vi "DataLib.pack data.vi"(1 "dataIn":T1, 2 "DAQDevice":string, 3 "Data Descriptor":T2, 4 "DAQDeviceData":T1) -> (15 "dataOut":T1)   [LabVIEW 2014, in "DataLib.lvlib"]
doc: "Packs the data of each DAQ device by the EventBuilder class."
uses:
  DataLib.lvlib
  CSCore/CSSystem/CoreDefs/CoreDefs.rawDataType.ctl
  CSCore/BaseProcess/BaseProcess.descriptor string definition.ctl
  CSCore/CSSystem/CoreLib/CoreLib.string 2 byte array.vi
  CSCore/CSSystem/CoreLib/CoreLib.lvlib
  CSCore/BaseProcess/BaseProcess.lvlib
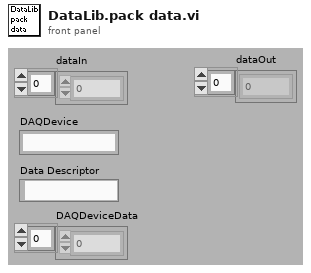
[diagram p1: front panel]
types:
  T1 = typedef "CoreDefs.rawDataType.ctl" = i8[]
  T2 = typedef "BaseProcess.lvlib/BaseProcess.descriptor string definition.ctl" = string
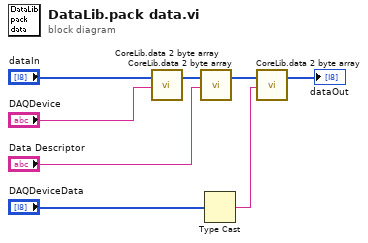
[diagram p0: block diagram]
diagram:
  n1 = call-poly "CoreLib.data 2 byte array.vi"("byteArray"="dataIn", "string"="DAQDevice") -> ("byteArray out"=w7:T1)  [unwired: 17 in]
  n2 = call-poly "CoreLib.data 2 byte array.vi"("byteArray"=w7, "string"="Data Descriptor") -> ("byteArray out"=w4:T1)  [unwired: 17 in]
  n3 = Type Cast(x="DAQDeviceData") -> (*(type *) &x=w1:string)  [unwired: 1 in]
  n4 = call-poly "CoreLib.data 2 byte array.vi"("byteArray"=w4, "string"=w1) -> ("byteArray out"=→"dataOut":T1)  [unwired: 17 in]
